vi "String(ms) to Stamp.vi"   [LabVIEW 2020]
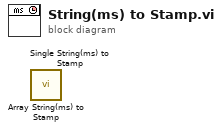
[diagram p0: block diagram]
diagram:
  n1 = call "Array String(ms) to Stamp.vi"() -> ()  [unwired: 5 in, 1 out]
  n2 = call "Single String(ms) to Stamp.vi"() -> ()  [unwired: 5 in, 1 out]
